vi "Read data file.vi"(11 "Application Directory":path) -> (0 "Graph data":cluster{"Array":dbl[], "Array":dbl[]}[](array[cluster]), 1 "Header":string, 2 "Mode":T1=enum."FD EPR", 3 "Name":string, 4 "Error Out":errorcluster)   [LabVIEW 2022 SP3]
uses:
  Datatypes/Measurement type.ctl
  <vilib>/Utility/error.llb/Error Cluster From Error Code.vi
  <vilib>/ErrorRing/Error Ring.xnode
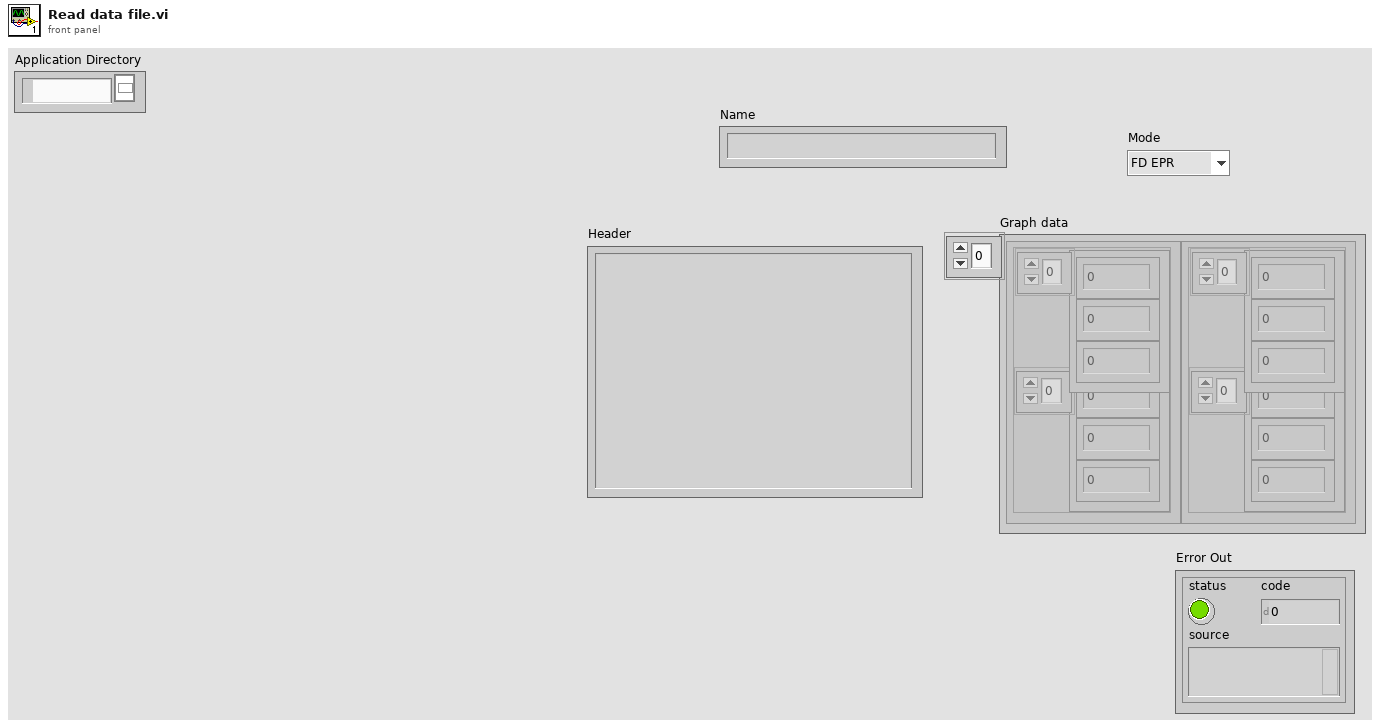
[diagram p1: front panel]
types:
  T1 = typedef "Measurement type.ctl" = enum16{"MD EPR", "FD EPR"}
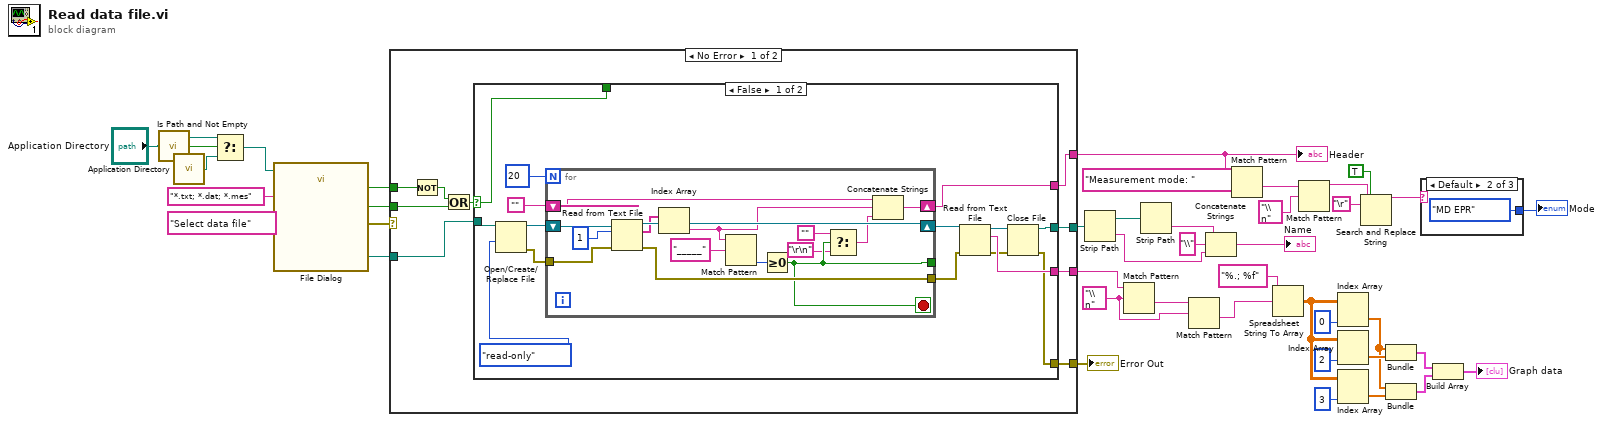
[diagram p0: block diagram]
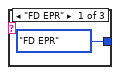
[diagram p2: hidden frame]
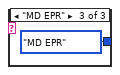
[diagram p3: hidden frame]
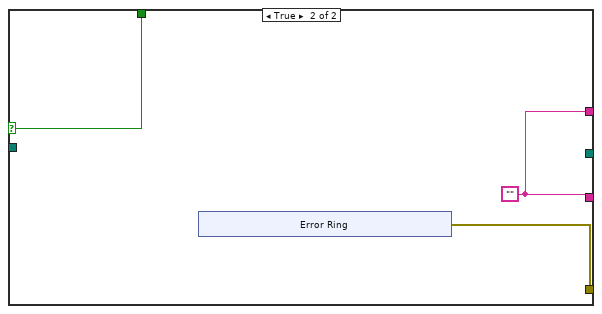
[diagram p4: hidden frame]
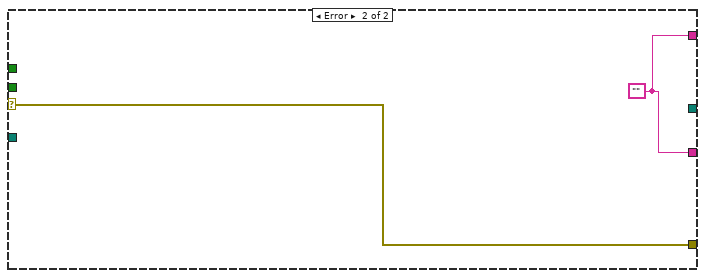
[diagram p5: hidden frame]
diagram:
  w1 = "\\n" ("regular expression")
  n1 = call <vilib>:"Is Path and Not Empty.vi"("path"="Application Directory") -> ("Is Path and Not Empty?"=w12:bool)  [unwired: 4 in]
  n2 = call <vilib>:"Application Directory.vi"() -> ("Application Directory"=w9:path)
  n3 = Select(t="Application Directory", s=w12, f=w9) -> (s? t:f=w10:path)
  n4 = call "File Dialog"("start path"=w10, "prompt"="Select data file", "pattern (all files)"="*.txt; *.dat; *.mes") -> ("selected path"=w40:path, "exists"=w39:bool, "cancelled"=w38:bool, "error out"=w37:errorcluster)  [unwired: 9 in]
  n5 = case shown="No Error" w37 {
    selector: w37 -> [_ w89]
    tunnel: w40 -> [w50 _]
    tunnel: w39 -> [w49 _]
    tunnel: w38 -> [w46 _]
    tunnel: [w45 w88] -> w16
    tunnel: [w44 w88] -> w29
    tunnel: [w43 _] -> w35
    tunnel: [w42 w89] -> w36
    frame No Error {
      n6 = Not(x=w49) -> (.not. x?=w48:bool)
      n7 = Or(x=w48, y=w46) -> (x .or. y?=w47:bool)
      n8 = case shown="False" w47 {
        selector: w47 -> [w65 w83]
        tunnel: w50 -> [w56 _]
        tunnel: [w65 w83] -> _
        tunnel: [w63 w81] -> w45
        tunnel: [w61 w81] -> w44
        tunnel: [w58 _] -> w43
        tunnel: [w51 w82] -> w42
        frame False {
          n9 = Open/Create/Replace File(file path (use dialog)=w56, access (0:read/write)=enum16{"read/write", "read-only", "write-only"}."read-only") -> (refnum out=w55:refnum<file>, error out=w53:errorcluster)  [unwired: 4 in, 1 out]
          n10 = for {
            N: 20 -> [_]
            shift-right: [w72] -> w63
            shift-left: "" -> [w70]
            tunnel: [w68] -> _
            shift-right: [w77] -> w62
            shift-left: w55 -> [w76]
            tunnel: [w75] -> w57
            tunnel: w53 -> [w74]
            stop <- w68 stop-if-true
            n11 = Read from Text File(file (use dialog)=w76, count=1, error in=w74) -> (refnum out=w77:refnum<file>, text=w73:string[], error out=w75:errorcluster)  [unwired: 1 in, 1 out]
            n12 = Index Array(array=w73) -> (element=w71:string)  [unwired: 1 in]
            n13 = Match Pattern(string=w71, regular expression="_____") -> (offset past match=w78:i32)  [unwired: 1 in, 3 out]
            n14 = Greater Or Equal To 0?(x=w78) -> (x >= 0?=w68:bool)
            n15 = Select(t="", s=w68, f="\r\n") -> (s? t:f=w66:string)
            n16 = Concatenate Strings(w70, w71, w66) -> (w72:string)
          }
          n17 = Read from Text File(file (use dialog)=w62, error in=w57) -> (refnum out=w60:refnum<file>, text=w61:string, error out=w59:errorcluster)  [unwired: 2 in, 1 out]
          n18 = Close File(refnum=w60, error in=w59) -> (path=w58:path, error out=w51:errorcluster)
        }
        frame True {
          w81 = ""
          n19 = xnode "Error Ring"() -> ("error out"=w82:errorcluster)
        }
      }
    }
    frame Error {
      w88 = ""
    }
  }
  "Header" <- w16
  "Error Out" <- w36
  n20 = Strip Path(path=w35) -> (stripped path=w34:path, name=w31:string)
  n21 = Match Pattern(string=w29, regular expression=w1) -> (after substring=w3:string)  [unwired: 1 in, 3 out]
  n22 = Strip Path(path=w34) -> (name=w32:string)  [unwired: 1 out]
  n23 = Match Pattern(string=w3, regular expression=w1) -> (after substring=w2:string)  [unwired: 1 in, 3 out]
  n24 = Concatenate Strings(w32, "\\" ("string"), w31) -> (→"Name":string)
  n25 = Match Pattern(string=w16, regular expression="Measurement mode: ") -> (after substring=w15:string)  [unwired: 1 in, 3 out]
  n26 = Spreadsheet String To Array(format string="%.; %f", spreadsheet string=w2) -> (array=w22:dbl[][])  [unwired: 2 in]
  n27 = Match Pattern(string=w15, regular expression="\\n") -> (before substring=w7:string)  [unwired: 1 in, 3 out]
  n28 = Index Array(array=w22, index (col)=0 ("disabled index (col)")) -> (element=w19:dbl[])  [unwired: 1 in]
  n29 = Index Array(array=w22, index (col)=2 ("disabled index (col)")) -> (element=w20:dbl[])  [unwired: 1 in]
  n30 = Index Array(array=w22, index (col)=3 ("disabled index (col)")) -> (element=w21:dbl[])  [unwired: 1 in]
  n31 = Search and Replace String(replace all?=TRUE ("replace all? (F)"), input string=w7, search string="\r") -> (result string=w5:string)  [unwired: 5 in, 3 out]
  n32 = Bundle(w19, w20) -> (w26:cluster{dbl[], dbl[]})  [unwired: 1 in]
  n33 = Bundle(w19, w21) -> (w27:cluster{dbl[], dbl[]})  [unwired: 1 in]
  n34 = case shown="Default" w5 {
    tunnel: [Measurement_type."FD EPR" ("Mode") Measurement_type."MD EPR" ("Mode") Measurement_type."MD EPR" ("Mode")] -> w14
    frame "FD EPR" {
    }
    frame Default {
    }
    frame "MD EPR" {
    }
  }
  "Mode" <- w14
  n35 = Build Array(w26, w27) -> (→"Graph data":cluster{dbl[], dbl[]}[])
